vi "Error - Unknown Parameter.vi"(8 "error in":errorcluster, 9 "parameter":string, 10 "state":string, 11 "queue":refnum<queue>) -> (0 "error out":errorcluster, 3 "queue out":refnum<queue>)   [LabVIEW 2021]
uses:
  <vilib>/Utility/error.llb/Error Cluster From Error Code.vi
  <vilib>/ErrorRing/Error Ring.xnode
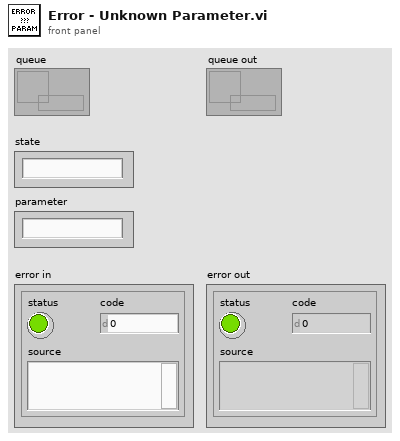
[diagram p1: front panel]
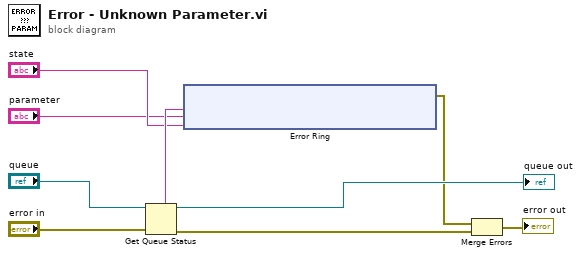
[diagram p0: block diagram]
diagram:
  n1 = Get Queue Status(queue="queue", error in (no error)="error in") -> (queue out=→"queue out":refnum<queue>, queue name=w3:string, error out=w4:errorcluster)  [unwired: 1 in, 5 out]
  n2 = xnode "Error Ring"("parameter 0"=w3, "parameter 1"="parameter", "parameter 2"="state") -> ("error out"=w5:errorcluster)
  n3 = Merge Errors(w5, w4) -> (→"error out":errorcluster)
